vi "IsPointInBounds.vi"(8 "error in (no error)":errorcluster, 10 "Point":dbl[](array[numeric]), 11 "object in":refnum<class "Zone.lvclass">) -> (0 "error out":errorcluster, 2 "InBounds":bool, 3 "object out":refnum<class "Zone.lvclass">)   [LabVIEW 2023, in "Zone.lvclass"]
uses:
  Zone.lvclass
  Zone.lvclass/Zone.ctl
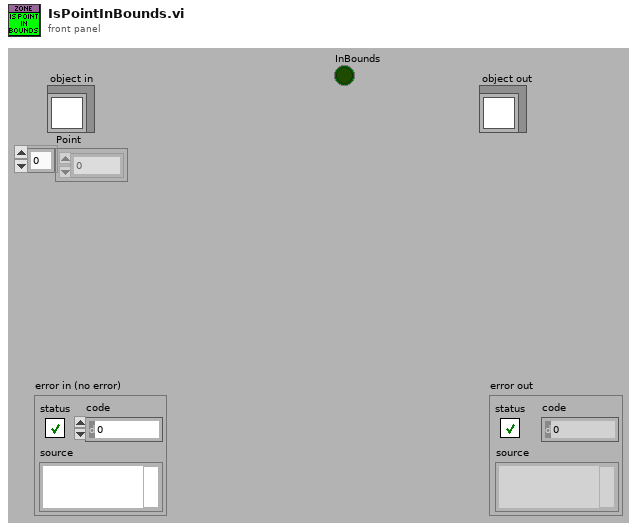
[diagram p1: front panel]
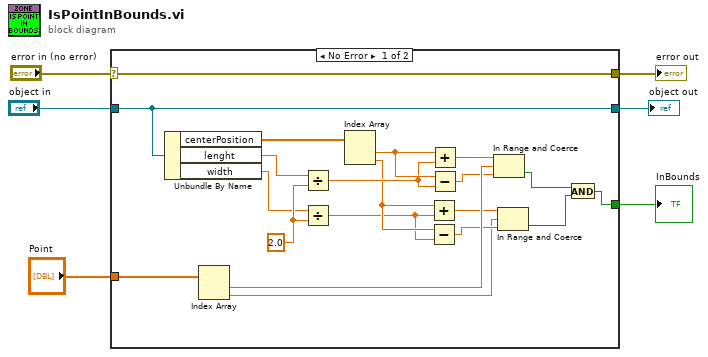
[diagram p0: block diagram]
diagram:
  n1 = case shown="No Error" "error in (no error)" {
    selector: "error in (no error)" -> [w26 w28]
    tunnel: [w26 w28] -> w5
    tunnel: [w25 w27] -> w3
    tunnel: "object in" -> [w25 w27]
    tunnel: "Point" -> [w20 _]
    tunnel: [w7 _] -> w1
    frame No Error {
      w23 = 2.0 ("y")
      n2 = Unbundle By Name(w25) -> ("centerPosition"=w21:dbl[], "lenght"=w24:dbl, "width"=w22:dbl)
      n3 = Index Array(array=w20) -> (element #1=w19:dbl, element #2=w12:dbl)  [unwired: 2 in]
      n4 = Divide(x=w24, y=w23) -> (x/y=w16:dbl)
      n5 = Divide(x=w22, y=w23) -> (x/y=w10:dbl)
      n6 = Index Array(array=w21) -> (element #1=w17:dbl, element #2=w11:dbl)  [unwired: 2 in]
      n7 = Add(x=w11, y=w10) -> (x+y=w14:dbl)
      n8 = Subtract(x=w11, y=w10) -> (x-y=w13:dbl)
      n9 = Add(x=w17, y=w16) -> (x+y=w18:dbl)
      n10 = Subtract(x=w17, y=w16) -> (x-y=w15:dbl)
      n11 = In Range and Coerce(upper limit=w18, x=w19, lower limit=w15) -> (In Range?=w9:bool)  [unwired: 1 out]
      n12 = In Range and Coerce(upper limit=w14, x=w12, lower limit=w13) -> (In Range?=w8:bool)  [unwired: 1 out]
      n13 = And(x=w9, y=w8) -> (x .and. y?=w7:bool)
    }
    frame Error {
    }
  }
  "error out" <- w5
  "object out" <- w3
  "InBounds" <- w1
